vi "ADO Command Set Stored Procedure Text.vi"(8 "error in (no error)":errorcluster, 9 "Prepare?":bool, 10 "CommandText":string, 11 "ADODB._Command In":refnum<k7>) -> (0 "error out":errorcluster, 3 "ADODB._Command Out":refnum<k7>)   [LabVIEW 2013]
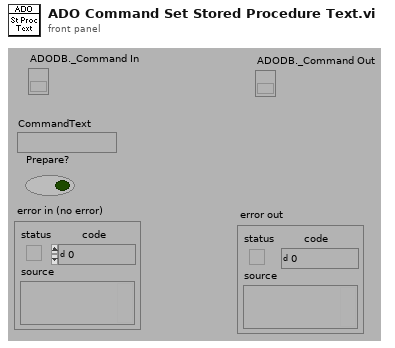
[diagram p1: front panel]
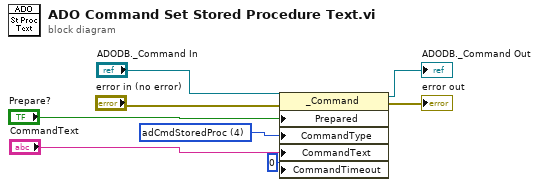
[diagram p0: block diagram]
diagram:
  w5 = 4 items=["adCmdUnspecified"=-1, "adCmdUnknown"=8, "adCmdText"=1, "adCmdTable"=2, "adCmdStoredProc"=4, "adCmdFile"=256, "adCmdTableDirect"=512] ("CommandType")
  n1 = property class="_Command"(reference="ADODB._Command In", error in="error in (no error)", "Prepared"="Prepare?", "CommandType"=w5, "CommandText"="CommandText", "CommandTimeout"=0) -> (reference out=→"ADODB._Command Out":refnum<k7>, error out=→"error out":errorcluster)
